vi "Sync DAC LMK04832.vi"(0 "fpga reference in":T7, 5 "board settings in":T1[](array[typedef]) {"Address Space" items=["VXI/VME A16"=1, "VXI/VME A24"=2, "VXI/VME A32"=3, "VXI/VME A64"=4, "PXI Memory Allocations"=9, "PXI Configuration"=10, "PXI BAR0"=11, "PXI BAR1"=12, "PXI BAR2"=13, "PXI BAR3"=14, "PXI BAR4"=15, "PXI BAR5"=16]}, 11 "error in":errorcluster) -> (6 "board settings out":T1[](array[typedef]) {"Address Space" items=["VXI/VME A16"=1, "VXI/VME A24"=2, "VXI/VME A32"=3, "VXI/VME A64"=4, "PXI Memory Allocations"=9, "PXI Configuration"=10, "PXI BAR0"=11, "PXI BAR1"=12, "PXI BAR2"=13, "PXI BAR3"=14, "PXI BAR4"=15, "PXI BAR5"=16]}, 15 "error out":errorcluster)   [LabVIEW 2019]
uses:
  TypeDefs/Shared FPGA Reference.ctl
  <instrlib>/niMmWave/ni3610 and ni3630/controls/public/Main Settings.ctl
  <vilib>/Instr/_visa.llb/VISA Register Access Address Space.ctl
  <instrlib>/niMmWave/ni3610 and ni3630/controls/public/Register Adresses.ctl
  <instrlib>/niMmWave/ni3610 and ni3630/controls/public/Base Card Type.ctl
  <instrlib>/niMmWave/ni3610 and ni3630/controls/private/IQ Card Revision.ctl
  <instrlib>/niMmWave/ni3610 and ni3630/controls/public/Board Capability.ctl
  <instrlib>/niMmWave/ni3610 and ni3630/controls/public/Trigger Sink.ctl
  <instrlib>/niMmWave/ni3610 and ni3630/controls/public/SPI Cmd.ctl
  <vilib>/Utility/error.llb/Error Cluster From Error Code.vi
  <vilib>/rvi/errors/niLvFpgaAdjustHostInterfaceError.vi
  <vilib>/rvi/interface/nirviReadWriteControl/nirviReadWriteControl.xnode
  <instrlib>/niMmWave/ni3610 and ni3630/ni3610_and_ni3630_Driver_Lib.lvlib
  NiFpgaLv.dll
  <vilib>/rvi/interface/Simulation/niFpgaSimulationCallBeginRW.vi
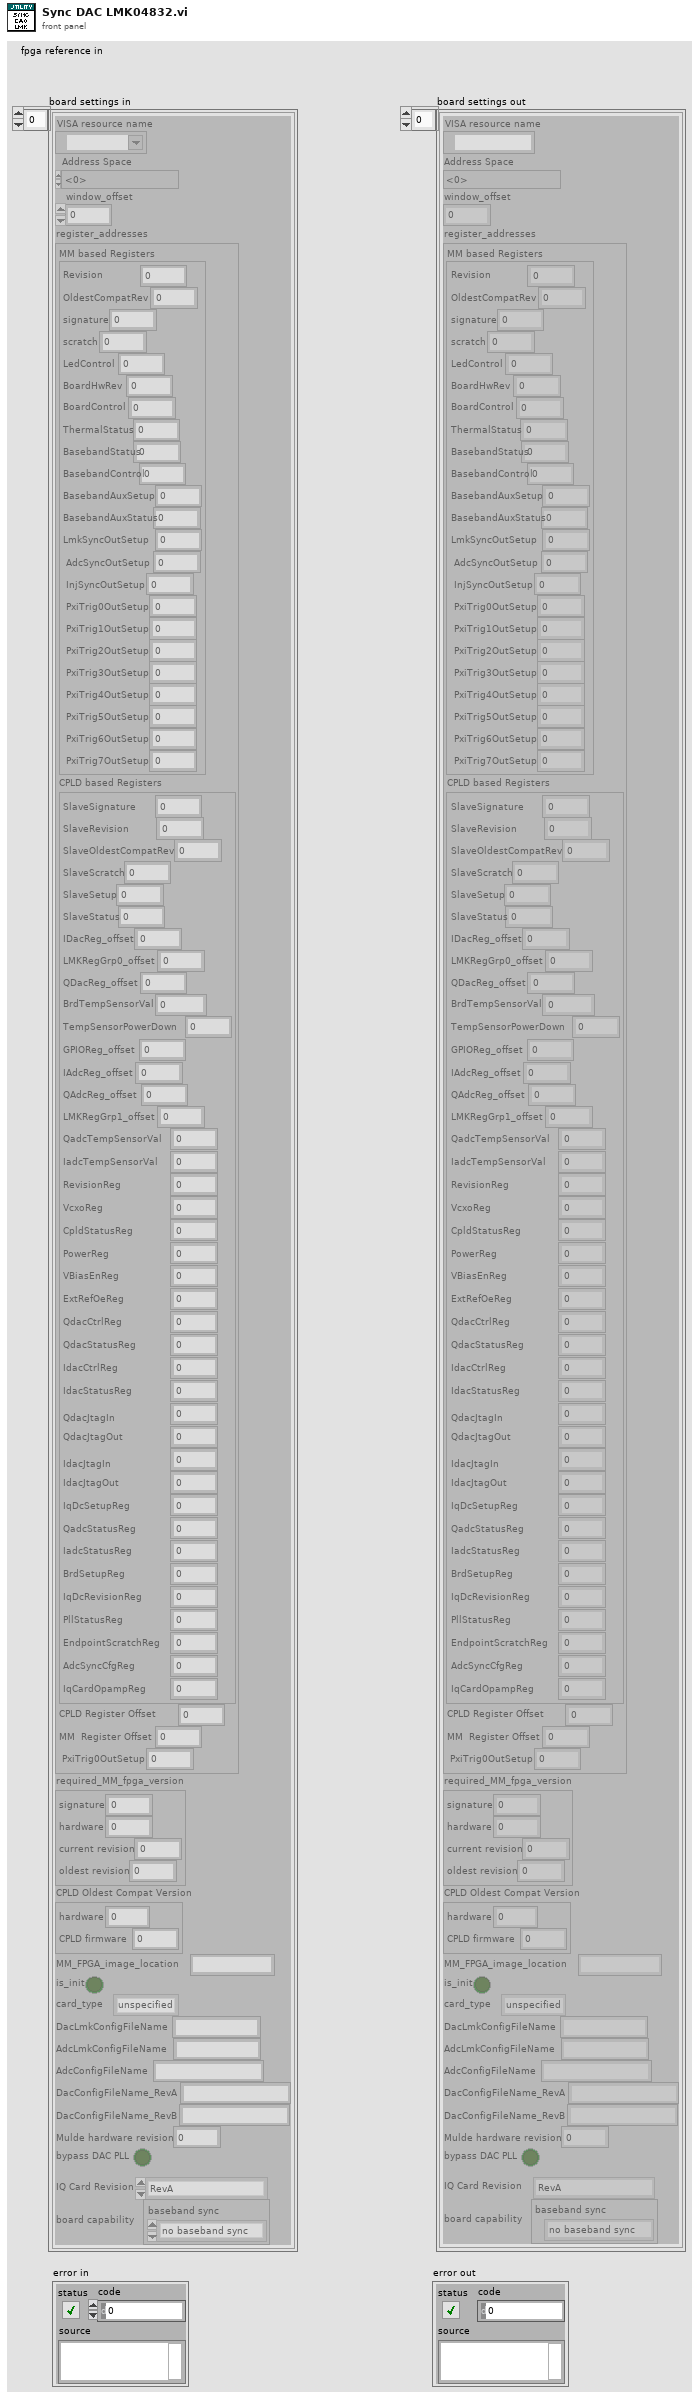
[diagram p1: front panel]
types:
  T1 = typedef "ni3610_and_ni3630_Driver_Lib.lvlib/Main Settings.ctl" = cluster{"VISA resource name":refnum<visa-resource-name>, "Address Space":T2, "window_offset":u32, "register_addresses":T3, "required_MM_fpga_version":cluster{"signature":u32, "hardware":u32, "current revision":u32, "oldest revision":u32}, "CPLD Oldest Compat Version ":cluster{"hardware":u32, "CPLD firmware":u32}, "MM_FPGA_image_location":string, "is_init":bool, "card_type":T4, "DacLmkConfigFileName":string, "AdcLmkConfigFileName":string, "AdcConfigFileName":string, "DacConfigFileName_RevA":string, "DacConfigFileName_RevB":string, "Mulde hardware revision":u8, "bypass DAC PLL\n":bool, "IQ Card Revision":T5, "board capability":T6}
  T2 = typedef "VISA Register Access Address Space.ctl" = u16
  T3 = typedef "ni3610_and_ni3630_Driver_Lib.lvlib/Register Adresses.ctl" = cluster{"MM based Registers":cluster{"Revision":u32, "OldestCompatRev":u32, "signature":u32, "scratch":u32, "LedControl":u32, "BoardHwRev":u32, "BoardControl":u32, "ThermalStatus":u32, "BasebandStatus":u32, "BasebandControl":u32, "BasebandAuxSetup":u32, "BasebandAuxStatus":u32, "LmkSyncOutSetup":u32, " AdcSyncOutSetup":u32, " InjSyncOutSetup":u32, " PxiTrig0OutSetup":u32, " PxiTrig1OutSetup":u32, " PxiTrig2OutSetup":u32, " PxiTrig3OutSetup":u32, " PxiTrig4OutSetup":u32, " PxiTrig5OutSetup":u32, " PxiTrig6OutSetup":u32, " PxiTrig7OutSetup":u32}, "CPLD based Registers":cluster{"SlaveSignature":u32, "SlaveRevision":u32, "SlaveOldestCompatRev":u32, "SlaveScratch":u32, "SlaveSetup":u32, "SlaveStatus":u32, "IDacReg_offset":u32, "LMKRegGrp0_offset":u32, "QDacReg_offset":u32, "BrdTempSensorVal":u32, "TempSensorPowerDown":u32, "GPIOReg_offset":u32, "IAdcReg_offset":u32, "QAdcReg_offset":u32, "LMKRegGrp1_offset":u32, "QadcTempSensorVal":u32, "IadcTempSensorVal":u32, "RevisionReg":u32, "VcxoReg":u32, "CpldStatusReg":u32, "PowerReg":u32, "VBiasEnReg":u32, "ExtRefOeReg":u32, "QdacCtrlReg":u32, "QdacStatusReg":u32, "IdacCtrlReg":u32, "IdacStatusReg":u32, "QdacJtagIn":u32, "QdacJtagOut":u32, "IdacJtagIn":u32, "IdacJtagOut":u32, "IqDcSetupReg":u32, "QadcStatusReg":u32, "IadcStatusReg":u32, "BrdSetupReg":u32, "IqDcRevisionReg":u32, "PllStatusReg":u32, "EndpointScratchReg":u32, "AdcSyncCfgReg":u32, "IqCardOpampReg":u32}, "CPLD Register Offset":u32, "MM  Register Offset":u32, " PxiTrig0OutSetup":u32}
  T4 = typedef "ni3610_and_ni3630_Driver_Lib.lvlib/Base Card Type.ctl" = enum16{"unspecified", "ADC", "DAC"}
  T5 = typedef "ni3610_and_ni3630_Driver_Lib.lvlib/IQ Card Revision.ctl" = enum16{"RevA", "RevB", "RevC", "RevD"}
  T6 = typedef "ni3610_and_ni3630_Driver_Lib.lvlib/Board Capability.ctl" = cluster{"baseband sync":enum16{"no baseband sync", "baseband sync"}}
  T7 = typedef "Shared FPGA Reference.ctl" = refnum<k20>
  T8 = typedef "ni3610_and_ni3630_Driver_Lib.lvlib/SPI Cmd.ctl" = cluster{"SPI address":u32, "SPI data":u32}
  T9 = typedef "ni3610_and_ni3630_Driver_Lib.lvlib/Trigger Sink.ctl" = enum16{"LmkSyncOutSetup", "AdcSyncOutSetup", "InjSyncOutSetup"}
  T10 = cluster{"control":cluster{"measure tdc":bool, "enable measurement":bool, "10 kHz tclk enable":bool, "200 kHz tclk enable":bool, "output enable":bool, "reset":bool, "deassert holdoff":u8, "calibrate":bool, "calibrate width":u8, "tclk trigger enable":bool, "alignment complete":bool}, "tclk parameters":cluster{"rollover count":u16, "rising edge count":u16, "falling edge count":u16}}
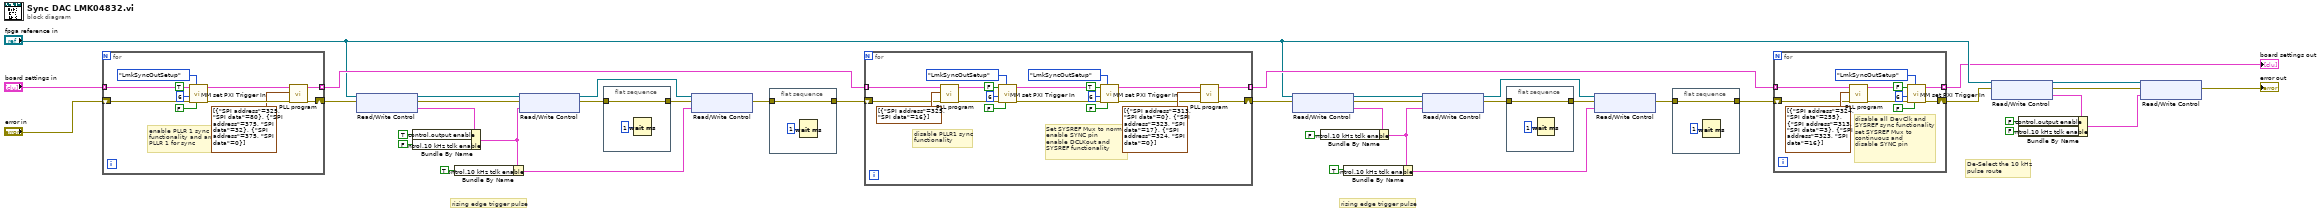
[diagram p0: block diagram]
diagram:
  # "De-Select the 10 kHz\npulse route"
  # "rising edge trigger pulse"
  # "rising edge trigger pulse"
  n1 = for {
    tunnel: "board settings in" -> [w47] mode=indexing
    shift-right: [w42] -> w30
    shift-left: "error in" -> [w46]
    tunnel: [w41] -> w27 mode=indexing
    # "enable PLLR 1 sync\nfunctionality and arm\nPLLR 1 for sync"
    n2 = call <instrlib>:"MM set PXI Trigger In.vi"("Force Enable"=FALSE, "Trigger Sink"=Trigger_Sink."LmkSyncOutSetup", "error in"=w46, "PXI Trigger Select (0..7)"=u8 6, "Enable Trigger Input"=TRUE, "Board Settings in"=w47) -> ("error out"=w44:errorcluster, "Board Settings out"=w43:T1)  [unwired: 4 in]
    n3 = call <instrlib>:"PLL program.vi"("error in"=w44, "SPI settings array"=T8[] [{"SPI address"=325, "SPI data"=80}, {"SPI address"=375, "SPI data"=32}, {"SPI address"=375, "SPI data"=0}], "Board Settings in"=w43) -> ("error out"=w42:errorcluster, "Board Settings out"=w41:T1)  [unwired: 7 in]
  }
  n4 = xnode "Read/Write Control"("FPGA VI Reference In"="fpga reference in", "error in"=w30) -> ("FPGA VI Reference Out"=w37:T7, "error out"=w2:errorcluster, "sync.parameters"=w34:T10)
  n5 = Bundle By Name(cluster=w34, "control.output enable"=TRUE, "control.10 kHz tclk enable"=FALSE ("control.pulse injection")) -> (w29:T10)
  n6 = Bundle By Name(cluster=w29, "control.10 kHz tclk enable"=TRUE ("control.measure")) -> (w16:T10)
  n7 = xnode "Read/Write Control"("FPGA VI Reference In"=w37, "error in"=w2, "sync.parameters"=w29) -> ("FPGA VI Reference Out"=w31:T7)  [unwired: 1 out]
  n8 = flat-sequence {
    tunnel: [w51] -> w28
    tunnel: w2 -> [w51]
    frame #0 {
      n9 = Wait (ms)(milliseconds to wait=u32 1) -> ()  [unwired: 1 out]
    }
  }
  n10 = xnode "Read/Write Control"("FPGA VI Reference In"=w31, "error in"=w28, "sync.parameters"=w16) -> ()  [unwired: 2 out]
  n11 = flat-sequence {
    tunnel: w28 -> [w52]
    tunnel: [w52] -> w13
    frame #0 {
      n12 = Wait (ms)(milliseconds to wait=u32 1) -> ()  [unwired: 1 out]
    }
  }
  n13 = for {
    shift-right: [w55] -> w18
    shift-left: w13 -> [w69]
    tunnel: [w54] -> w17 mode=indexing
    tunnel: w27 -> [w65] mode=indexing
    # "Set SYSREF Mux to normal\nenable SYNC pin\nenable DCLKout and\nSYSREF functionality"
    # "disable PLLR1 sync\nfunctionality"
    n14 = call <instrlib>:"PLL program.vi"("error in"=w69, "SPI settings array"=T8[] [{"SPI address"=325, "SPI data"=16}], "Board Settings in"=w65) -> ("error out"=w68:errorcluster, "Board Settings out"=w67:T1)  [unwired: 7 in]
    n15 = call <instrlib>:"MM set PXI Trigger In.vi"("Force Enable"=FALSE, "Trigger Sink"=Trigger_Sink."LmkSyncOutSetup", "error in"=w68, "PXI Trigger Select (0..7)"=u8 6, "Enable Trigger Input"=FALSE, "Board Settings in"=w67) -> ("error out"=w56:errorcluster, "Board Settings out"=w57:T1)  [unwired: 4 in]
    n16 = call <instrlib>:"MM set PXI Trigger In.vi"("Force Enable"=FALSE, "Trigger Sink"=Trigger_Sink."LmkSyncOutSetup", "error in"=w56, "PXI Trigger Select (0..7)"=u8 6, "Enable Trigger Input"=TRUE, "Board Settings in"=w57) -> ("error out"=w61:errorcluster, "Board Settings out"=w62:T1)  [unwired: 4 in]
    n17 = call <instrlib>:"PLL program.vi"("error in"=w61, "SPI settings array"=T8[] [{"SPI address"=313, "SPI data"=0}, {"SPI address"=323, "SPI data"=17}, {"SPI address"=324, "SPI data"=0}], "Board Settings in"=w62) -> ("error out"=w55:errorcluster, "Board Settings out"=w54:T1)  [unwired: 7 in]
  }
  n18 = xnode "Read/Write Control"("FPGA VI Reference In"="fpga reference in", "error in"=w18) -> ("FPGA VI Reference Out"=w20:T7, "error out"=w15:errorcluster, "sync.parameters"=w21:T10)
  n19 = Bundle By Name(cluster=w21, "control.10 kHz tclk enable"=FALSE ("control.measure")) -> (w23:T10)
  n20 = Bundle By Name(cluster=w23, "control.10 kHz tclk enable"=TRUE ("control.measure")) -> (w24:T10)
  n21 = xnode "Read/Write Control"("FPGA VI Reference In"=w20, "error in"=w15, "sync.parameters"=w23) -> ("FPGA VI Reference Out"=w22:T7, "error out"=w14:errorcluster)
  n22 = flat-sequence {
    tunnel: [w75] -> w25
    tunnel: w14 -> [w75]
    frame #0 {
      n23 = Wait (ms)(milliseconds to wait=u32 1) -> ()  [unwired: 1 out]
    }
  }
  n24 = xnode "Read/Write Control"("FPGA VI Reference In"=w22, "error in"=w25, "sync.parameters"=w24) -> ()  [unwired: 2 out]
  n25 = flat-sequence {
    tunnel: w25 -> [w76]
    tunnel: [w76] -> w26
    frame #0 {
      n26 = Wait (ms)(milliseconds to wait=u32 1) -> ()  [unwired: 1 out]
    }
  }
  n27 = for {
    shift-right: [w80] -> w10
    shift-left: w26 -> [w84]
    tunnel: [w81] -> w4 mode=indexing
    tunnel: w17 -> [w78] mode=indexing
    # "disable all DevClk and\nSYSREF sync functionality\nset SYSREF Mux to\ncontinuous and\ndisable SYNC pin"
    n28 = call <instrlib>:"PLL program.vi"("error in"=w84, "SPI settings array"=T8[] [{"SPI address"=324, "SPI data"=255}, {"SPI address"=313, "SPI data"=3}, {"SPI address"=323, "SPI data"=16}], "Board Settings in"=w78) -> ("error out"=w83:errorcluster, "Board Settings out"=w82:T1)  [unwired: 7 in]
    n29 = call <instrlib>:"MM set PXI Trigger In.vi"("Force Enable"=FALSE, "Trigger Sink"=Trigger_Sink."LmkSyncOutSetup", "error in"=w83, "PXI Trigger Select (0..7)"=u8 6, "Enable Trigger Input"=FALSE, "Board Settings in"=w82) -> ("error out"=w80:errorcluster, "Board Settings out"=w81:T1)  [unwired: 4 in]
  }
  "board settings out" <- w4
  n30 = xnode "Read/Write Control"("FPGA VI Reference In"="fpga reference in", "error in"=w10) -> ("FPGA VI Reference Out"=w7:T7, "error out"=w6:errorcluster, "sync.parameters"=w11:T10)
  n31 = Bundle By Name(cluster=w11, "control.output enable"=FALSE ("control.measure"), "control.10 kHz tclk enable"=FALSE ("control.tclk trigger enable")) -> (w5:T10)
  n32 = xnode "Read/Write Control"("FPGA VI Reference In"=w7, "error in"=w6, "sync.parameters"=w5) -> ("error out"=→"error out":errorcluster)  [unwired: 1 out]
